vi "Three Chart Temple.vi"(8 "error in (no error)":errorcluster caption="错误输入（无错误）") -> (0 "error out":errorcluster caption="错误输出")   [LabVIEW 2015]
doc: "该连续测量范例项目在队列消息处理器模板的基础上实现。\n\n事件处理循环负责按用户界面操作生成对应的消息。\n\n消息处理循环负责对事件处理循环或其他消息生成的消息进行处理。其中还包括用于采集和记录消息处理循环的子VI，以及用于更新图表的循环。"
uses:
  Settings/Settings.ctl
  Acquisition/Hardware Configuration.ctl
  Logging/Logging Configuration.ctl
  Motor Control/Hardware Configuration.ctl
  controls/UI Data.ctl
  controls/UI State.ctl
  support/Message Queue/Enqueue Message (Single).vi
  <vilib>/Utility/error.llb/Error Cluster From Error Code.vi
  <vilib>/ErrorRing/Error Ring.xnode
  Acquisition/Acquisition.lvlib
  Logging/Logging.lvlib
  Settings/Settings.lvlib
  support/User Event - Stop/User Event - Stop.lvlib
  support/Message Queue/Message Queue.lvlib
  Motor Control/Motor Control.lvlib
panel:
  out "XY Graph":cluster{"Y":dbl[], "Y":dbl[]}[](graph) caption="XY图"
  out "XY Graph 2":cluster{"Y":dbl[], "Y":dbl[]}[](graph) caption="XY图"
  out "XY Graph 3":cluster{"Y":dbl[], "Y":dbl[]}[](graph) caption="XY图"
  in  "清零":bool
  in  "读取":bool
  out "模拟通道5":dbl
  out "模拟通道4":dbl
  out "模拟通道3":dbl
  out "模拟通道2":dbl
  out "模拟通道1":dbl
  out "模拟通道0":dbl
  out "角度":dbl
  in  "计算":bool
  in  "Start":bool caption="开始"
  in  "Stop":bool caption="停止"
  out "Status":string caption="状态"
  in  "Exit":bool caption="退出"
  # "测量项目"
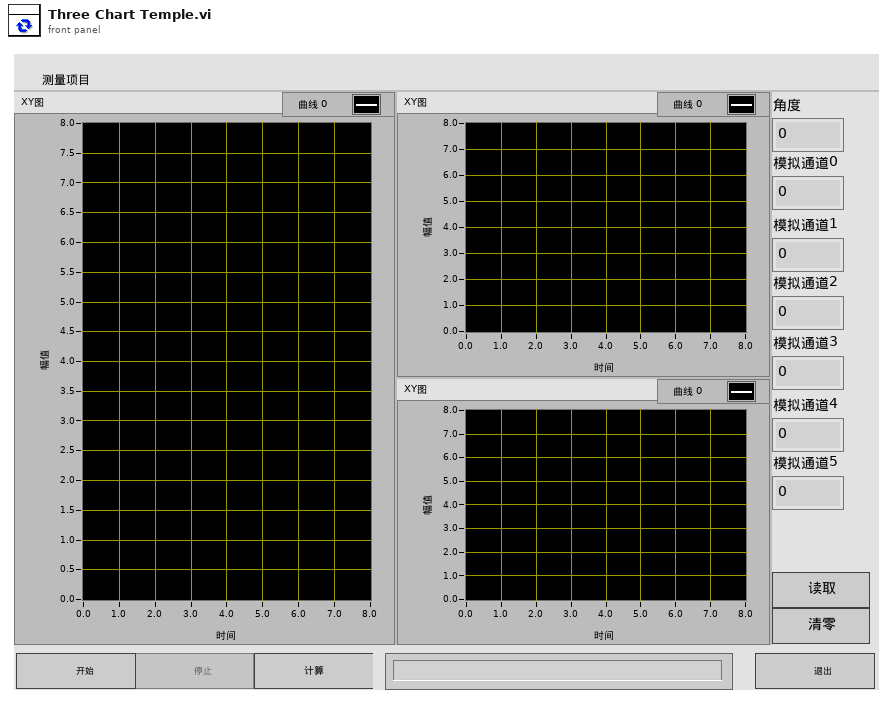
[diagram p1: front panel]
types:
  T1 = typedef "Motor Control.lvlib/电机转动逻辑1.ctl" = cluster{"反转判断条件1":T2, "停止判断条件1":T3}
  T2 = typedef "Motor Control.lvlib/反转判断条件1.ctl" = cluster{"传感器序号":i32, "条件":enum16{"小于", "大于", "等于"}, "值":dbl, "条件判断时间间隔":i32}
  T3 = typedef "Motor Control.lvlib/停止判断条件1.ctl" = cluster{"角度传感器序号":i32, "正转/反转":enum16{"正转", "反转"}, "反转次数":i32, "停止角度":dbl, "停止角度误差范围":dbl}
  T4 = typedef "UI State.ctl" = enum16{"Idle", "Acquiring and Logging", "Waiting for Exit", "Waiting for Exit (Acq Stopped)", "Waiting for Exit (Log Stopped)", "Waiting for Stop", "Waiting for Stop (Acq Stopped)", "Waiting for Stop (Log Stopped)"}
  T5 = typedef "UI Data.ctl" = cluster{"Start Ref":refnum<vi>, "Stop Ref":refnum<vi>, "calculate Ref":refnum<vi>, "Status Ref":refnum<vi>, "Exit Ref":refnum<vi>, "Data Ref":refnum<vi>, "read Ref":refnum<vi>, "clean Ref":refnum<vi>}
  T6 = typedef "Settings.lvlib/Settings.ctl" = cluster{"Hardware Configuration":T7, "Logging Configuration":T8, "电机设置":T9, "啮合测试电机转动逻辑":T1, "功能测试电机转动逻辑":T1, "力提特性电机转动逻辑":T1}
  T7 = typedef "Acquisition.lvlib/Hardware Configuration.ctl" = cluster{"电压读取设置":cluster{"DAQmx Channel":tag, "Max Input":dbl, "Min Input":dbl, "Sample Rate":dbl, "Sample Number":i32, "DAQmx Task":refnum<k21>}, "角度传感器设置":cluster{"counter":tag, "units":i32, "分辨率":i32, "初始角度":dbl, "DecodingType":i32, "A相端口":tag, "B相端口":tag, "task in":refnum<k21>}}
  T8 = typedef "Logging.lvlib/Logging Configuration.ctl" = cluster{"Log File Base Path":path, "电压传感器转换率":dbl[], "电压传感器本底":dbl[]}
  T9 = typedef "Motor Control.lvlib/Hardware Configuration.ctl" = cluster{"counter":tag, "方向端口":tag, "当前方向":bool, "频率":dbl, "DAQmx Task":refnum<k21>}
  T10 = typedef "Message Queue.lvlib/All Message Queues.ctl" = cluster{"UI":refnum<queue>, "Acquisition":refnum<queue>, "Logging":refnum<queue>, "MotorCtrl":refnum<queue>, "plot logic":refnum<queue>}
  T11 = typedef "Logging.lvlib/计算类型.ctl" = enum16{"啮合", "退回", "功能", "力特性"}
  T12 = enum8{"Enabled", "Disabled", "Disabled and Grayed Out"}
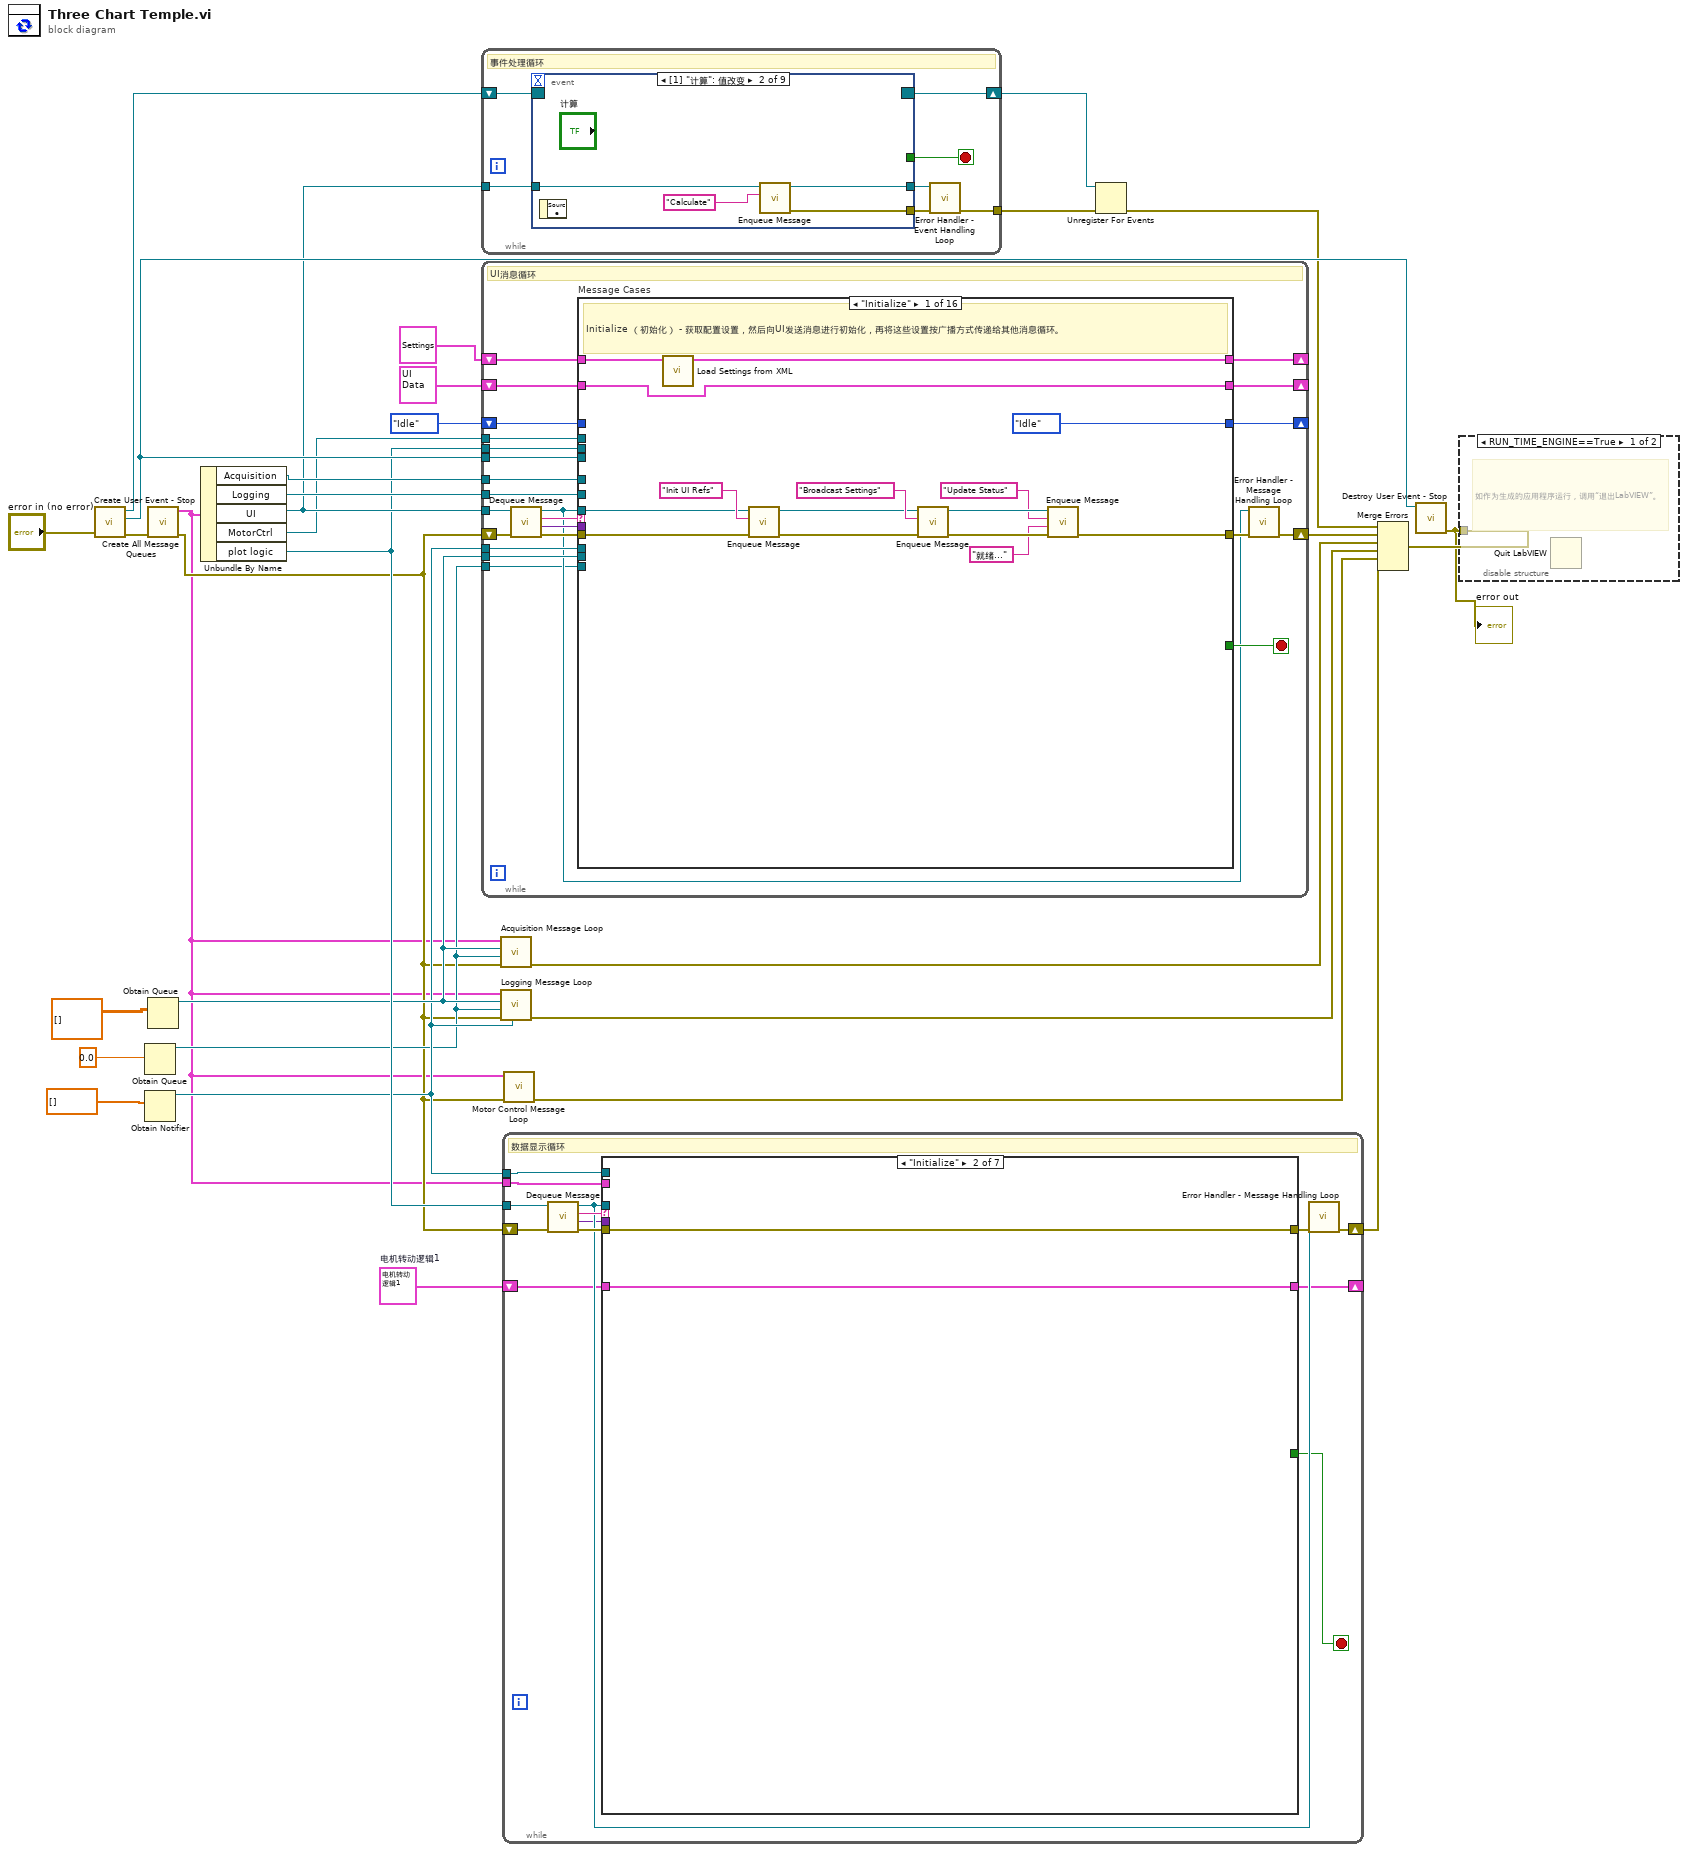
[diagram p0: block diagram]
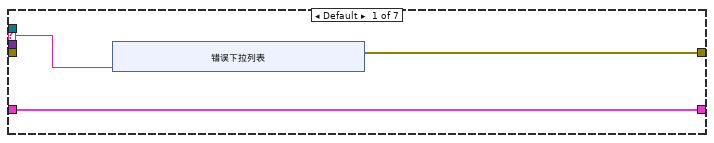
[diagram p3: hidden frame]
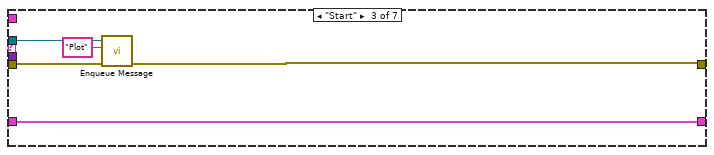
[diagram p4: hidden frame]
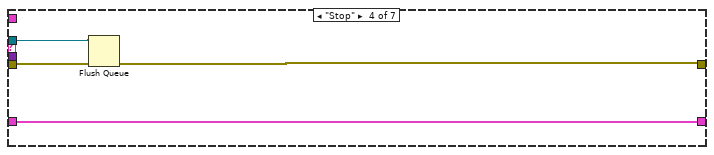
[diagram p5: hidden frame]
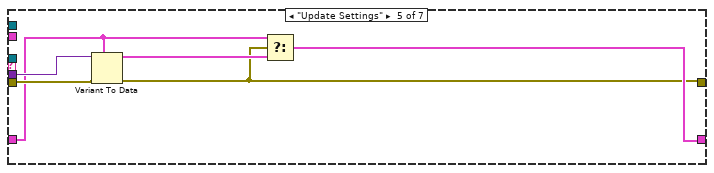
[diagram p6: hidden frame]
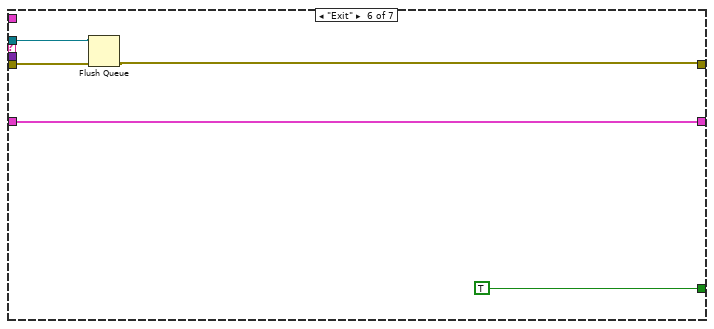
[diagram p7: hidden frame]
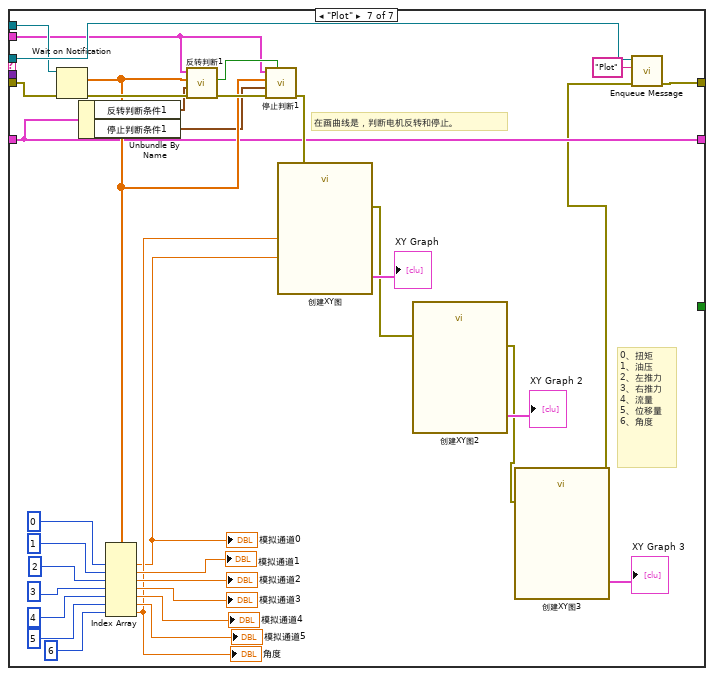
[diagram p8: hidden frame]
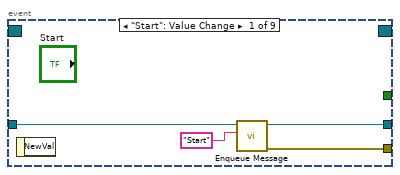
[diagram p9: hidden frame]
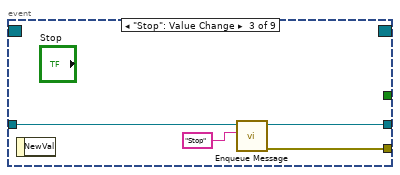
[diagram p10: hidden frame]
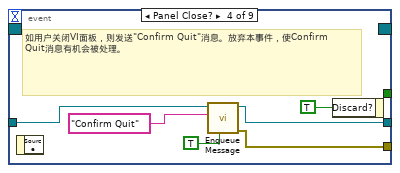
[diagram p11: hidden frame]
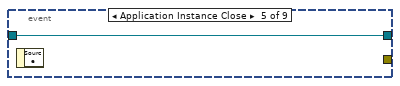
[diagram p12: hidden frame]
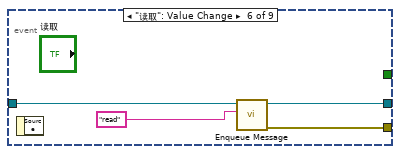
[diagram p13: hidden frame]
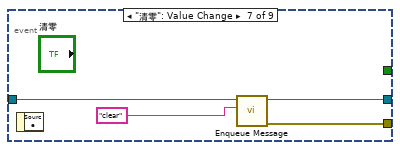
[diagram p14: hidden frame]
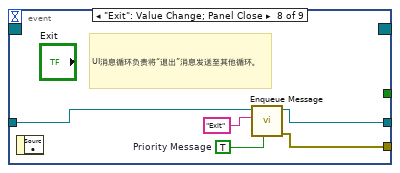
[diagram p15: hidden frame]
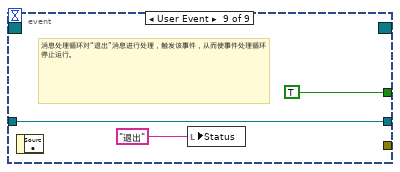
[diagram p16: hidden frame]
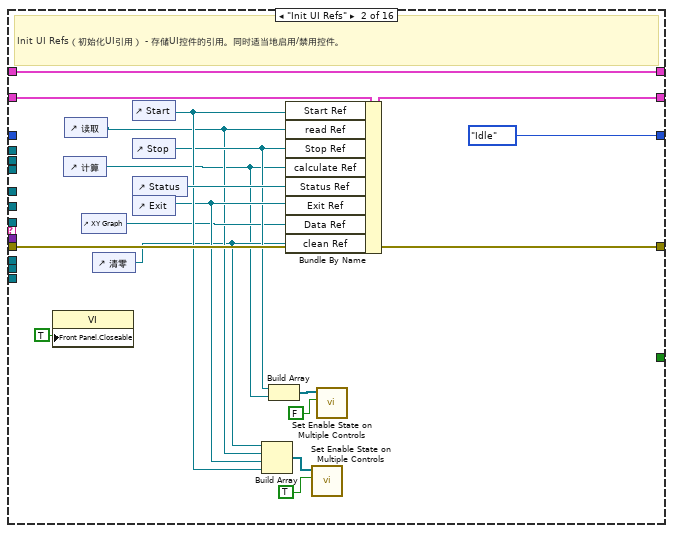
[diagram p17: hidden frame]
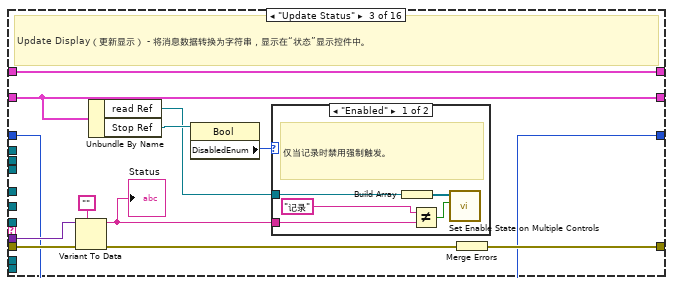
[diagram p18: hidden frame]
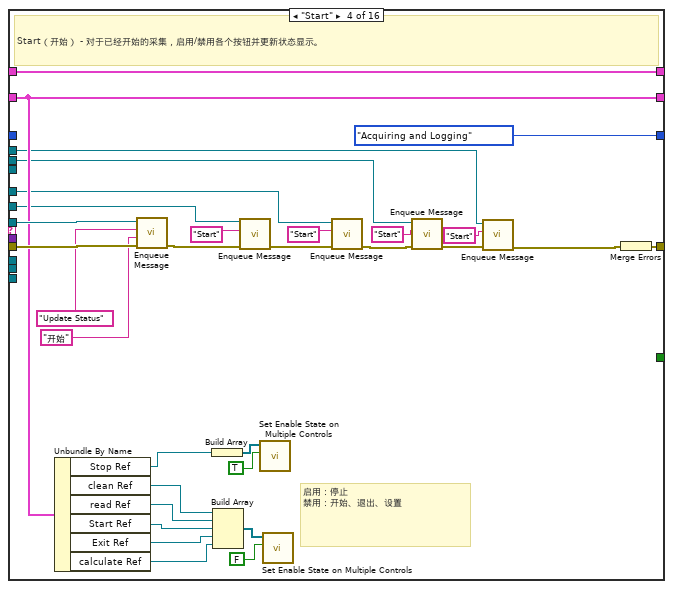
[diagram p20: hidden frame]
diagram:
  w3 = T1 {"反转判断条件1"={"传感器序号"=0, "条件"=enum."小于", "值"=0.0, "条件判断时间间隔"=0}, "停止判断条件1"={"角度传感器序号"=0, "正转/反转"=enum."正转", "反转次数"=0, "停止角度"=0.0, "停止角度误差范围"=0.0}}  # 电机转动逻辑1
  n1 = call "Create User Event - Stop.vi"("error in (no error)"="error in (no error)") -> ("error out"=w25:errorcluster, "User Event - Stop"=w27:refnum<user-event>, "Stop Event Registration Refnum"=w28:refnum<event-registration>)  [unwired: 8 in]
  n2 = Obtain Queue(element data type=0.0) -> (queue out=w8:refnum<queue>)  [unwired: 4 in, 2 out]
  n3 = Obtain Notifier(notification data type=dbl[] []) -> (notifier out=w10:refnum<notifier>)  [unwired: 3 in, 2 out]
  n4 = call "Create All Message Queues.vi"("error in (no error)"=w25) -> ("error out"=w7:errorcluster, "Message Queues out"=w4:T10)  [unwired: 9 in]
  n5 = Obtain Queue(element data type=dbl[][] []) -> (queue out=w11:refnum<queue>)  [unwired: 4 in, 2 out]
  n6 = Unbundle By Name(w4) -> ("Acquisition"=w19:refnum<queue>, "Logging"=w18:refnum<queue>, "UI"=w17:refnum<queue>, "MotorCtrl"=w15:refnum<queue>, "plot logic"=w14:refnum<queue>)
  n7 = while {
    tunnel: w17 -> [w37]
    tunnel: [w32] -> w30
    shift-right: [w36] -> w21
    shift-left: w28 -> [w38]
    stop <- w35 stop-if-true
    # "事件处理循环"
    n8 = event shown="[1] \"计算\": 值改变" {
      selector: w38 -> [_ _ _ _ _ _ _ _ _]
      dyn-events: [_ _ _ _ _ _ _ _ _] -> w36
      timeout: _ -> [_ _ _ _ _ _ _ _ _]
      tunnel: [_ _ _ _ _ _ _ _ TRUE ("Discard?")] -> w35
      tunnel: w37 -> [w40 w45 w49 w56 w57 w59 w63 w67 w71]
      tunnel: [w42 w44 w48 w51 _ w61 w65 w70 _] -> w33
      tunnel: [w39 w43 w47 w52 w57 w58 w62 w66 w71] -> w34
      event "Start": Value Change {
        n9 = event-data() -> ()  [unwired: 1 in, 1 out]
        n10 = call-poly "Enqueue Message.vi"("Message"="Start", "Message Queue"=w40) -> ("error out"=w42:errorcluster, "dup Message Queue"=w39:refnum<queue>)  [unwired: 8 in]
      }
      event "计算": Value Change {
        n11 = event-data() -> ()  [unwired: 1 in, 1 out]
        n12 = call-poly "Enqueue Message.vi"("Message"="Calculate", "Message Queue"=w45) -> ("error out"=w44:errorcluster, "dup Message Queue"=w43:refnum<queue>)  [unwired: 8 in]
      }
      event "Stop": Value Change {
        n13 = event-data() -> ()  [unwired: 1 in, 1 out]
        n14 = call-poly "Enqueue Message.vi"("Message"="Stop", "Message Queue"=w49) -> ("error out"=w48:errorcluster, "dup Message Queue"=w47:refnum<queue>)  [unwired: 8 in]
      }
      event Panel Close? {
        # "如用户关闭VI面板，则发送\"Confirm Quit\"消息。放弃本事件，使Confirm Quit消息有机会被处理。"
        n15 = event-data() -> ()  [unwired: 1 in, 1 out]
        n16 = call-poly "Enqueue Message.vi"("Priority Message? (F)"=TRUE, "Message"="Confirm Quit", "Message Queue"=w56) -> ("error out"=w51:errorcluster, "dup Message Queue"=w52:refnum<queue>)  [unwired: 7 in]
        n17 = event-data("Discard?"=TRUE) -> ()  [unwired: 1 in, 1 out]
      }
      event Application Instance Close {
        n18 = event-data() -> ()  [unwired: 1 in, 1 out]
      }
      event "读取": Value Change {
        n19 = event-data() -> ()  [unwired: 1 in, 1 out]
        n20 = call-poly "Enqueue Message.vi"("Message"="read", "Message Queue"=w59) -> ("error out"=w61:errorcluster, "dup Message Queue"=w58:refnum<queue>)  [unwired: 8 in]
      }
      event "清零": Value Change {
        n21 = event-data() -> ()  [unwired: 1 in, 1 out]
        n22 = call-poly "Enqueue Message.vi"("Message"="clear", "Message Queue"=w63) -> ("error out"=w65:errorcluster, "dup Message Queue"=w62:refnum<queue>)  [unwired: 8 in]
      }
      event "Exit": Value Change; Panel Close {
        w68 = TRUE  # Priority Message
        # "UI消息循环负责将“退出”消息发送至其他循环。"
        n23 = event-data() -> ()  [unwired: 1 in, 1 out]
        n24 = call-poly "Enqueue Message.vi"("Priority Message? (F)"=w68, "Message"="Exit", "Message Queue"=w67) -> ("error out"=w70:errorcluster, "dup Message Queue"=w66:refnum<queue>)  [unwired: 7 in]
      }
      event User Event {
        # "消息处理循环对“退出”消息进行处理，触发该事件，从而使事件处理循环停止运行。"
        n25 = event-data() -> ()  [unwired: 1 in, 1 out]
        n26 = local write "Status"("退出" ("Exit String")) -> ()
      }
    }
    n27 = call "Error Handler - Event Handling Loop.vi"("error in (no error)"=w33, "Message Queue"=w34) -> ("dup error in"=w32:errorcluster)  [unwired: 8 in, 1 out]
  }
  n28 = while {
    tunnel: w17 -> [w90]
    tunnel: w27 -> [w95]
    shift-right: [w80] -> w31
    shift-left: w7 -> [w94]
    shift-right: [w89] -> _
    shift-left: T6 {"Hardware Configuration"={"电压读取设置"={"DAQmx Channel"="", "Max Input"=0.0, "Min Input"=0.0, "Sample Rate"=0.0, "Sample Number"=0, "DAQmx Task"=""}, "角度传感器设置"={"counter"="Dev1/ctr0", "units"=10146, "分辨率"=0, "初始角度"=0.0, "DecodingType"=10092, "A相端口"="/Dev1/PFI8", "B相端口"="/Dev1/PFI8", "task in"=""}}, "Logging Configuration"={"Log File Base Path"=path "", "电压传感器转换率"=[], "电压传感器本底"=[]}, "电机设置"={"counter"="Dev1/ctr0", "方向端口"="", "当前方向"=FALSE, "频率"=0.0, "DAQmx Task"=""}, "啮合测试电机转动逻辑"={"反转判断条件1"={"传感器序号"=0, "条件"=enum."小于", "值"=0.0, "条件判断时间间隔"=0}, "停止判断条件1"={"角度传感器序号"=0, "正转/反转"=enum."正转", "反转次数"=0, "停止角度"=0.0, "停止角度误差范围"=0.0}}, "功能测试电机转动逻辑"={"反转判断条件1"={"传感器序号"=0, "条件"=enum."小于", "值"=0.0, "条件判断时间间隔"=0}, "停止判断条件1"={"角度传感器序号"=0, "正转/反转"=enum."正转", "反转次数"=0, "停止角度"=0.0, "停止角度误差范围"=0.0}}, "力提特性电机转动逻辑"={"反转判断条件1"={"传感器序号"=0, "条件"=enum."小于", "值"=0.0, "条件判断时间间隔"=0}, "停止判断条件1"={"角度传感器序号"=0, "正转/反转"=enum."正转", "反转次数"=0, "停止角度"=0.0, "停止角度误差范围"=0.0}}} ("Settings") -> [w88]
    shift-right: [w86] -> _
    shift-left: T5 {"Start Ref"=refnum, "Stop Ref"=refnum, "calculate Ref"=refnum, "Status Ref"=refnum, "Exit Ref"=refnum, "Data Ref"=refnum, "read Ref"=refnum, "clean Ref"=refnum} ("Measurement UI Controls") -> [w87]
    tunnel: w19 -> [w85]
    tunnel: w18 -> [w84]
    tunnel: w10 -> [w83]
    tunnel: w11 -> [w82]
    shift-right: [w77] -> _
    shift-left: UI_State."Idle" ("UI State") -> [w78]
    tunnel: w15 -> [w74]
    tunnel: w14 -> [w75]
    tunnel: w8 -> [w76]
    stop <- w96 stop-if-true
    # "UI消息循环"
    n29 = call "Dequeue Message.vi"("error in (no error)"=w94, "Message Queue"=w90) -> ("error out"=w93:errorcluster, "Message Data"=w91:variant, "Message"=w92:string, "dup Message Queue"=w79:refnum<queue>)  [unwired: 6 in]
    n30 = case "Message Cases" shown="\"Initialize\"" w92 {
      selector: w92 -> [_ _ _ _ _ _ _ _ _ _ _ _ _ _ _ w381]
      tunnel: w79 -> [w101 _ _ w176 _ w216 w220 w245 _ w293 w308 w318 w356 _ _ _]
      tunnel: w93 -> [w100 w129 w140 w175 w182 w215 w222 w247 w270 w295 w312 w317 w363 w370 w375 _]
      tunnel: [w107 w129 w141 w177 w185 w217 w221 w246 w287 w290 w303 w316 w364 w369 w379 w382] -> w81
      tunnel: [_ _ _ _ _ _ _ _ _ _ _ _ TRUE _ _ _] -> w96
      tunnel: w91 -> [_ _ w139 _ _ _ _ _ _ _ w311 _ _ _ _ _]
      tunnel: w95 -> [_ _ _ _ _ _ _ _ _ _ _ _ w362 _ _ _]
      tunnel: [w110 w128 w136 w174 w184 w214 w226 w251 w285 w292 w314 w321 w360 w368 w378 w384] -> w89
      tunnel: w88 -> [w111 w128 w136 w174 w184 w214 w226 w251 w285 w296 w314 w321 w360 w368 w378 w384]
      tunnel: w87 -> [w103 w127 w135 w171 w183 w211 w225 w250 w282 w289 w313 w320 w359 w367 w377 w383]
      tunnel: [w103 w126 w135 w171 w183 w211 w225 w250 w282 w289 w313 w320 w359 w367 w377 w383] -> w86
      tunnel: w85 -> [_ _ _ w159 _ w199 _ _ w281 _ _ _ w358 _ _ _]
      tunnel: w84 -> [_ _ _ w161 w179 w202 _ _ w280 _ _ _ w357 _ w373 _]
      tunnel: w83 -> [_ _ _ _ _ _ _ _ _ _ _ _ w355 _ _ _]
      tunnel: w82 -> [_ _ _ _ _ _ _ _ _ _ _ _ w352 _ _ _]
      tunnel: w78 -> [_ _ w130 _ w178 w197 w224 w249 w279 w288 w302 w319 _ w366 w376 w380]
      tunnel: [UI_State."Idle" ("UI State") UI_State."Idle" ("UI State") w130 UI_State."Acquiring and Logging" ("UI State") w178 w196 w223 w248 w279 w288 w302 w315 UI_State."Idle" ("UI State") w366 w376 w380] -> w77
      tunnel: w76 -> [_ _ _ _ _ _ _ _ _ _ _ _ w347 _ _ _]
      tunnel: w75 -> [_ _ _ w153 _ w189 _ _ w274 _ _ _ w346 _ _ _]
      tunnel: w74 -> [_ _ _ w149 _ w187 _ _ w277 _ _ _ w345 _ _ _]
      frame "Initialize" {
        # "Initialize （初始化） - 获取配置设置，然后向UI发送消息进行初始化，再将这些设置按广播方式传递给其他消息循环。"
        n31 = call "Load Settings from XML.vi"("Settings in"=w111) -> ("Settings out"=w110:T6)  [unwired: 9 in, 1 out]
        n32 = call-poly "Enqueue Message.vi"("error in (no error)"=w100, "Message"="Init UI Refs", "Message Queue"=w101) -> ("error out"=w98:errorcluster, "dup Message Queue"=w99:refnum<queue>)  [unwired: 7 in]
        n33 = call-poly "Enqueue Message.vi"("error in (no error)"=w98, "Message"="Broadcast Settings", "Message Queue"=w99) -> ("error out"=w109:errorcluster, "dup Message Queue"=w108:refnum<queue>)  [unwired: 7 in]
        n34 = call-poly "Enqueue Message.vi"("error in (no error)"=w109, "Message Data"="就绪..." ("Ready..."), "Message"="Update Status", "Message Queue"=w108) -> ("error out"=w107:errorcluster)  [unwired: 6 in, 1 out]
      }
      frame "Init UI Refs" {
        # "Init UI Refs（初始化UI引用） - 存储UI控件的引用。同时适当地启用/禁用控件。"
        n35 = property class="VI"("Front Panel.Closeable"=TRUE ("Front Panel Window:Closeable")) -> ()  [unwired: 2 in, 2 out]
        n36 = control-ref of="计算"() -> (w112:refnum<vi>)
        n37 = control-ref of="读取"() -> (w114:refnum<vi>)
        n38 = control-ref of="XY Graph"() -> (w115:refnum<vi>)
        n39 = control-ref of="清零"() -> (w113:refnum<vi>)
        n40 = control-ref of="Start"() -> (w122:refnum<vi>)
        n41 = control-ref of="Stop"() -> (w118:refnum<vi>)
        n42 = control-ref of="Status"() -> (w123:refnum<vi>)
        n43 = control-ref of="Exit"() -> (w119:refnum<vi>)
        n44 = Build Array(w113, w114, w119, w122) -> (w121:refnum<vi>[])
        n45 = Build Array(w118, w112) -> (w117:refnum<vi>[])
        n46 = Bundle By Name(cluster=w127, "Start Ref"=w122, "read Ref"=w114, "Stop Ref"=w118, "calculate Ref"=w112, "Status Ref"=w123, "Exit Ref"=w119, "Data Ref"=w115, "clean Ref"=w113) -> (w126:T5)
        n47 = call "Set Enable State on Multiple Controls.vi"("Enable?"=TRUE, "Controls"=w121) -> ()  [unwired: 10 in]
        n48 = call "Set Enable State on Multiple Controls.vi"("Enable?"=FALSE, "Controls"=w117) -> ()  [unwired: 10 in]
      }
      frame "Update Status" {
        # "Update Display（更新显示） - 将消息数据转换为字符串，显示在“状态”显示控件中。"
        n49 = Variant To Data(error in=w140, type="", Variant=w139) -> (data=w132:string, error out=w137:errorcluster)
        "Status" <- w132
        n50 = Unbundle By Name(w135) -> ("read Ref"=w131:refnum<vi>, "Stop Ref"=w134:refnum<vi>)
        n51 = property class="Bool"(reference=w134) -> ("DisabledEnum"=w133:T12)  [unwired: 1 in, 2 out]
        n52 = case shown="\"Enabled\"" w133 {
          tunnel: w132 -> [w144 _]
          tunnel: w131 -> [w145 _]
          frame "Enabled" {
            # "仅当记录时禁用强制触发。"
            n53 = Build Array(w145) -> (w146:refnum<vi>[])
            n54 = Not Equal?(x="记录" ("Logging"), y=w144) -> (x != y?=w142:bool)
            n55 = call "Set Enable State on Multiple Controls.vi"("Enable?"=w142, "Controls"=w146) -> ()  [unwired: 10 in]
          }
          frame "Disabled", Default {
          }
        }
        n56 = Merge Errors(w137) -> (w141:errorcluster)
      }
      frame "Start" {
        # "启用：停止\n禁用：开始、退出、设置"
        # "Start（开始） - 对于已经开始的采集，启用/禁用各个按钮并更新状态显示。"
        n57 = Unbundle By Name(w171) -> ("Stop Ref"=w154:refnum<vi>, "clean Ref"=w155:refnum<vi>, "read Ref"=w156:refnum<vi>, "Start Ref"=w166:refnum<vi>, "Exit Ref"=w165:refnum<vi>, "calculate Ref"=w164:refnum<vi>)
        n58 = call-poly "Enqueue Message.vi"("error in (no error)"=w175, "Message Data"="开始" ("Waiting for trigger"), "Message"="Update Status", "Message Queue"=w176) -> ("error out"=w163:errorcluster)  [unwired: 6 in, 1 out]
        n59 = Build Array(w154) -> (w168:refnum<vi>[])
        n60 = Build Array(w155, w156, w166, w165, w164) -> (w169:refnum<vi>[])
        n61 = call-poly "Enqueue Message.vi"("error in (no error)"=w163, "Message"="Start", "Message Queue"=w161) -> ("error out"=w160:errorcluster)  [unwired: 7 in, 1 out]
        n62 = call "Set Enable State on Multiple Controls.vi"("Enable?"=TRUE, "Controls"=w168) -> ()  [unwired: 10 in]
        n63 = call "Set Enable State on Multiple Controls.vi"("Enable?"=FALSE, "Controls"=w169) -> ()  [unwired: 10 in]
        n64 = call-poly "Enqueue Message.vi"("error in (no error)"=w160, "Message"="Start", "Message Queue"=w159) -> ("error out"=w151:errorcluster)  [unwired: 7 in, 1 out]
        n65 = call-poly "Enqueue Message.vi"("error in (no error)"=w151, "Message"="Start", "Message Queue"=w153) -> ("error out"=w150:errorcluster)  [unwired: 7 in, 1 out]
        n66 = call-poly "Enqueue Message.vi"("error in (no error)"=w150, "Message"="Start", "Message Queue"=w149) -> ("error out"=w147:errorcluster)  [unwired: 7 in, 1 out]
        n67 = Merge Errors(w147) -> (w177:errorcluster)
      }
      frame "Force Trigger" {
        # "Force Trigger（强制触发） - 发送消息至记录消息循环，开始记录。"
        n68 = call-poly "Enqueue Message.vi"("error in (no error)"=w182, "Message"="Force Trigger", "Message Queue"=w179) -> ("error out"=w181:errorcluster)  [unwired: 7 in, 1 out]
        n69 = Merge Errors(w181) -> (w185:errorcluster)
      }
      frame "Stop" {
        # "停止画图、电机、记录，最后停止采集。"
        # "启用：开始、退出、设置\n禁用：停止"
        # "停止－对于已经停止的采集，启用/禁用各个按钮并更新状态显示。"
        n70 = Unbundle By Name(w211) -> ("Stop Ref"=w193:refnum<vi>, "read Ref"=w194:refnum<vi>, "clean Ref"=w195:refnum<vi>, "Start Ref"=w206:refnum<vi>, "Exit Ref"=w205:refnum<vi>, "calculate Ref"=w204:refnum<vi>)
        n71 = call-poly "Enqueue Message.vi"("error in (no error)"=w215, "Message Data"="就绪..." ("Ready..."), "Message"="Update Status", "Message Queue"=w216) -> ("error out"=w192:errorcluster)  [unwired: 6 in, 1 out]
        n72 = Build Array(w194, w195, w206, w205, w204) -> (w209:refnum<vi>[])
        n73 = Build Array(w193) -> (w208:refnum<vi>[])
        n74 = call "Set Enable State on Multiple Controls.vi"("Enable?"=TRUE, "Controls"=w209) -> ()  [unwired: 10 in]
        n75 = call "Set Enable State on Multiple Controls.vi"("Enable?"=FALSE, "Controls"=w208) -> ()  [unwired: 10 in]
        n76 = call-poly "Enqueue Message.vi"("error in (no error)"=w192, "Message"="Stop", "Message Queue"=w189) -> ("error out"=w191:errorcluster)  [unwired: 7 in, 1 out]
        n77 = call-poly "Enqueue Message.vi"("error in (no error)"=w191, "Message"="Stop", "Message Queue"=w187) -> ("error out"=w190:errorcluster)  [unwired: 7 in, 1 out]
        n78 = call-poly "Enqueue Message.vi"("error in (no error)"=w190, "Message"="Stop", "Message Queue"=w202) -> ("error out"=w201:errorcluster)  [unwired: 7 in, 1 out]
        n79 = case shown="默认" w197 {
          selector: w197 -> [_ w219]
          tunnel: [UI_State."Waiting for Stop" ("UI State") w219] -> w196
          frame Default {
          }
          frame "Waiting for Exit" {
          }
        }
        n80 = call-poly "Enqueue Message.vi"("error in (no error)"=w201, "Message"="Stop", "Message Queue"=w199) -> ("error out"=w200:errorcluster)  [unwired: 7 in, 1 out]
        n81 = Merge Errors(w200) -> (w217:errorcluster)
      }
      frame "Acquisition Stopped" {
        # "此处代码用于确定采集停止时采取何种操作。"
        n82 = case shown="\"Waiting for Stop (Log Stopped)\"" w224 {
          selector: w224 -> [w228 _ _ _ _]
          tunnel: [w228 UI_State."Waiting for Exit (Acq Stopped)" ("UI State") UI_State."Waiting for Stop (Acq Stopped)" ("UI State") UI_State."Idle" ("UI State") UI_State."Idle" ("UI State")] -> w223
          tunnel: w222 -> [w227 w229 w231 w237 w243]
          tunnel: [w227 w229 w231 w236 w242] -> w221
          tunnel: w220 -> [_ _ _ w235 w241]
          frame Default {
          }
          frame "Waiting for Exit", "Waiting for Exit (Acq Stopped)" {
          }
          frame "Waiting for Stop", "Waiting for Stop (Acq Stopped)" {
          }
          frame "Waiting for Exit (Log Stopped)" {
            # "如果正在等待退出且记录已结束，“采集停止”消息表示应退出。"
            n83 = call-poly "Enqueue Message.vi"("Priority Message? (F)"=TRUE, "error in (no error)"=w237, "Message"="Exit", "Message Queue"=w235) -> ("error out"=w236:errorcluster)  [unwired: 6 in, 1 out]
          }
          frame "Waiting for Stop (Log Stopped)" {
            # "当前状态为等待停止时，如已停止记录，则收到\"Acquisition Stopped\"消息时即可停止。"
            n84 = call-poly "Enqueue Message.vi"("error in (no error)"=w243, "Message Data"="Ready..." ("Message"), "Message"="Update Status", "Message Queue"=w241) -> ("error out"=w242:errorcluster)  [unwired: 6 in, 1 out]
          }
        }
      }
      frame "Logging Stopped" {
        # "此处代码用于确定记录停止时采取何种操作。"
        n85 = case shown="\"Waiting for Stop (Acq Stopped)\"" w249 {
          selector: w249 -> [w253 _ _ _ _]
          tunnel: [w253 UI_State."Waiting for Exit (Log Stopped)" ("UI State") UI_State."Waiting for Stop (Log Stopped)" ("UI State") UI_State."Idle" ("UI State") UI_State."Idle" ("UI State")] -> w248
          tunnel: w247 -> [w252 w254 w256 w262 w268]
          tunnel: [w252 w254 w256 w261 w267] -> w246
          tunnel: w245 -> [_ _ _ w260 w266]
          frame Default {
          }
          frame "Waiting for Exit", "Waiting for Exit (Log Stopped)" {
          }
          frame "Waiting for Stop", "Waiting for Stop (Log Stopped)" {
          }
          frame "Waiting for Exit (Acq Stopped)" {
            # "如果正在等待退出且采集已结束，“记录停止”消息表示应退出。"
            n86 = call-poly "Enqueue Message.vi"("Priority Message? (F)"=TRUE, "error in (no error)"=w262, "Message"="Exit", "Message Queue"=w260) -> ("error out"=w261:errorcluster)  [unwired: 6 in, 1 out]
          }
          frame "Waiting for Stop (Acq Stopped)" {
            # "如果正在等待停止且采集已结束，“记录停止”消息表示应停止。"
            n87 = call-poly "Enqueue Message.vi"("error in (no error)"=w268, "Message Data"="Ready..." ("Message"), "Message"="Update Status", "Message Queue"=w266) -> ("error out"=w267:errorcluster)  [unwired: 6 in, 1 out]
          }
        }
      }
      frame "Broadcast settings" {
        w273 = "Update Settings" ("Message")
        # "向“记录和采集”消息队列发送“更新设置”消息。"
        n88 = Unbundle By Name(w285) -> ("Hardware Configuration"=w284:T7, "Logging Configuration"=w283:T8, "电机设置"=w276:T9, "啮合测试电机转动逻辑"=w272:T1)
        n89 = call-poly "Enqueue Message.vi"("error in (no error)"=w270, "Message Data"=w284, "Message"=w273, "Message Queue"=w281) -> ("error out"=w286:errorcluster)  [unwired: 6 in, 1 out]
        n90 = call-poly "Enqueue Message.vi"("error in (no error)"=w286, "Message Data"=w283, "Message"=w273, "Message Queue"=w280) -> ("error out"=w278:errorcluster)  [unwired: 6 in, 1 out]
        n91 = call-poly "Enqueue Message.vi"("error in (no error)"=w278, "Message Data"=w276, "Message"=w273, "Message Queue"=w277) -> ("error out"=w275:errorcluster)  [unwired: 6 in, 1 out]
        n92 = call-poly "Enqueue Message.vi"("error in (no error)"=w275, "Message Data"=w272, "Message"=w273, "Message Queue"=w274) -> ("error out"=w271:errorcluster)  [unwired: 6 in, 1 out]
        n93 = Merge Errors(w271, w270) -> (w287:errorcluster)
      }
      frame "Launch Settings Dialog" {
        # "用户单击“设置”按钮时，启动设置对话框。"
        n94 = call "Settings Dialog.vi"("error in (no error)"=w295, "Settings in"=w296) -> ("error out"=w291:errorcluster, "Cancelled?"=w294:bool, "Settings out"=w292:T6)  [unwired: 6 in, 1 out]
        n95 = case shown="假" w294 {
          tunnel: w293 -> [w300 _]
          tunnel: w291 -> [w299 w301]
          tunnel: [w298 w301] -> w290
          frame False {
            n96 = call-poly "Enqueue Message.vi"("error in (no error)"=w299, "Message"="Broadcast Settings", "Message Queue"=w300) -> ("error out"=w298:errorcluster)  [unwired: 7 in, 1 out]
          }
          frame True {
          }
        }
      }
      frame "Error" {
        # "Error - 检查错误消息数据及其响应。该消息由应用程序各循环结束处的“错误处理”VI发送。"
        n97 = Variant To Data(error in=w312, type=errorcluster {"status"=FALSE, "code"=0, "source"=""} ("error out"), Variant=w311) -> (data=w309:errorcluster, error out=w305:errorcluster)
        n98 = call <vilib>:"Simple Error Handler.vi"("error in (no error)"=w309) -> ()  [unwired: 4 in, 5 out]
        n99 = call-poly "Enqueue Message.vi"("Priority Message? (F)"=TRUE, "Message"="Exit", "Message Queue"=w308) -> ("error out"=w304:errorcluster)  [unwired: 7 in, 1 out]
        n100 = Merge Errors(w304, w305) -> (w303:errorcluster)
      }
      frame "Confirm Quit" {
        # "Confirm Quit - 该消息用于确认用户是否需要退出应用程序。"
        n101 = case shown="\"Acquiring and Logging\"" w319 {
          tunnel: w318 -> [w326 w332]
          tunnel: w317 -> [w325 w330]
          tunnel: [w322 w329] -> w316
          tunnel: [UI_State."Idle" ("UI State") w328] -> w315
          frame Default {
            # "如收到'Confirm Quit'消息时系统处于空闲状态，则不需要弹出确认提示。"
            n102 = call-poly "Enqueue Message.vi"("Priority Message? (F)"=TRUE, "error in (no error)"=w325, "Message"="Exit", "Message Queue"=w326) -> ("error out"=w322:errorcluster)  [unwired: 6 in, 1 out]
          }
          frame "Acquiring and Logging" {
            n103 = Two Button Dialog(message="采集仍在执行中，是否确定退出？" ("Confirm Quit Message"), 1:"否" ("No"), 2:"是" ("Yes")) -> (T button?=w331:bool)
            n104 = case shown="真" w331 {
              tunnel: w332 -> [_ w342]
              tunnel: w330 -> [w336 w341]
              tunnel: [w336 w340] -> w329
              tunnel: [UI_State."Acquiring and Logging" ("UI State") UI_State."Waiting for Exit" ("UI State")] -> w328
              frame False {
                # "用户不希望退出。"
              }
              frame True {
                n105 = call-poly "Enqueue Message.vi"("error in (no error)"=w341, "Message"="Stop", "Message Queue"=w342) -> ("error out"=w340:errorcluster)  [unwired: 7 in, 1 out]
              }
            }
          }
        }
      }
      frame "Exit" {
        w343 = TRUE ("Priority Message? (F)")
        w344 = "Exit" ("Message")
        # "不必检查错误输出。采集和记录队列可能已被释放。"
        # "停止VI。"
        # "Exit（退出）－触发用户事件，使“事件处理”循环停止运行。同时向“采集和记录”循环发送“退出”消息。"
        n106 = Release Queue(queue=w356, error in (no error)=w363) -> (error out=w354:errorcluster)  [unwired: 1 in, 2 out]
        n107 = call "Fire User Event - Stop.vi"("User Event - Stop"=w362) -> ("error out"=w361:errorcluster)  [unwired: 10 in]
        n108 = Release Notifier(notifier=w355, error in (no error)=w354) -> (error out=w353:errorcluster)  [unwired: 1 in, 2 out]
        n109 = Release Queue(queue=w352, error in (no error)=w353) -> (error out=w349:errorcluster)  [unwired: 1 in, 2 out]
        n110 = call-poly "Enqueue Message.vi"("Priority Message? (F)"=TRUE, "Message"=w344, "Message Queue"=w358) -> ()  [unwired: 7 in, 2 out]
        n111 = Release Queue(queue=w347, error in (no error)=w349) -> (error out=w348:errorcluster)  [unwired: 1 in, 2 out]
        n112 = call-poly "Enqueue Message.vi"("Priority Message? (F)"=w343, "Message"=w344, "Message Queue"=w357) -> ()  [unwired: 7 in, 2 out]
        n113 = call-poly "Enqueue Message.vi"("Priority Message? (F)"=w343, "Message"=w344, "Message Queue"=w346) -> ()  [unwired: 7 in, 2 out]
        n114 = call-poly "Enqueue Message.vi"("Priority Message? (F)"=w343, "Message"=w344, "Message Queue"=w345) -> ()  [unwired: 7 in, 2 out]
        n115 = Merge Errors(w361, w348) -> (w364:errorcluster)
      }
      frame "---Copy This Frame---" {
        # "如需创建新消息，可创建该帧的副本。在副本中，将本注释更改为对应消息的注释。"
        n116 = Merge Errors(w370) -> (w369:errorcluster)
      }
      frame "Calculate" {
        # "发指令让记录线程执行计算，传入相应的计算类型。"
        # "如需创建新消息，可创建该帧的副本。在副本中，将本注释更改为对应消息的注释。"
        n117 = call-poly "Enqueue Message.vi"("error in (no error)"=w375, "Message Data"=计算类型."啮合" ("计算类型"), "Message"="Calculate", "Message Queue"=w373) -> ("error out"=w374:errorcluster)  [unwired: 6 in, 1 out]
        n118 = Merge Errors(w374) -> (w379:errorcluster)
      }
      frame Default {
        # "如得到的消息未经任何分支定义，则运行“默认”分支。输出程序错误。"
        n119 = xnode "错误下拉列表"("参数 0"=w381) -> ("错误输出"=w382:errorcluster)
      }
    }
    n120 = call "Error Handler - Message Handling Loop.vi"("error in (no error)"=w81, "Message Queue"=w79) -> ("dup error in"=w80:errorcluster)  [unwired: 8 in, 1 out]
  }
  n121 = call "Acquisition Message Loop.vi"("error in (no error)"=w7, "Angle Data Queue"=w8, "Analog Data Queue"=w11, "Message Queues"=w4) -> ("error out"=w26:errorcluster)  [unwired: 7 in]
  n122 = call "Logging Message Loop.vi"("数据通知器"=w10, "error in (no error)"=w7, "Angle Data Queue"=w8, "Analog Data Queue"=w11, "Message Queues"=w4) -> ("error out"=w24:errorcluster)  [unwired: 6 in]
  n123 = while "Data Display Loop" {
    tunnel: w10 -> [w397]
    tunnel: w14 -> [w404]
    shift-right: [w399] -> w5
    shift-left: w7 -> [w403]
    tunnel: w4 -> [w395]
    shift-right: [w392] -> _
    shift-left: w3 -> [w393]
    stop <- w396 stop-if-true
    # "数据显示循环"
    n124 = call "Dequeue Message.vi"("error in (no error)"=w403, "Message Queue"=w404) -> ("error out"=w401:errorcluster, "Message Data"=w394:variant, "Message"=w400:string, "dup Message Queue"=w398:refnum<queue>)  [unwired: 6 in]
    n125 = case shown="\"Initialize\"" w400 {
      selector: w400 -> [w406 _ _ _ _ _ _]
      tunnel: [w407 w415 w418 w424 w426 w434 w453] -> w402
      tunnel: w401 -> [_ w415 w421 w425 w430 w436 w467]
      tunnel: w398 -> [_ _ w420 w423 _ w435 w470]
      tunnel: w397 -> [_ _ _ _ _ _ w468]
      tunnel: [_ _ _ _ _ TRUE _] -> w396
      tunnel: w395 -> [_ _ _ _ _ _ w447]
      tunnel: w394 -> [_ _ _ _ w429 _ _]
      tunnel: [w405 w416 w417 w422 w427 w432 w444] -> w392
      tunnel: w393 -> [w405 w416 w417 w422 w428 w432 w444]
      frame Default {
        n126 = xnode "错误下拉列表"("参数 0"=w406) -> ("错误输出"=w407:errorcluster)
      }
      frame "Initialize" {
      }
      frame "Start" {
        n127 = call-poly "Enqueue Message.vi"("error in (no error)"=w421, "Message"="Plot", "Message Queue"=w420) -> ("error out"=w418:errorcluster)  [unwired: 7 in, 1 out]
      }
      frame "Stop" {
        n128 = Flush Queue(queue=w423, error in (no error)=w425) -> (error out=w424:errorcluster)  [unwired: 2 out]
      }
      frame "Update Settings" {
        n129 = Variant To Data(error in=w430, type=w428, Variant=w429) -> (data=w431:T1, error out=w426:errorcluster)
        n130 = Select(t=w428, s=w426, f=w431) -> (s? t:f=w427:T1)
      }
      frame "Exit" {
        n131 = Flush Queue(queue=w435, error in (no error)=w436) -> (error out=w434:errorcluster)  [unwired: 2 out]
      }
      frame "Plot" {
        # "在画曲线是，判断电机反转和停止。"
        # "0、扭矩\n1、油压\n2、左推力\n3、右推力\n4、流量\n5、位移量\n6、角度"
        n132 = Wait on Notification(notifier=w468, error in (no error)=w467) -> (notification=w446:dbl[], error out=w450:errorcluster)  [unwired: 2 in, 2 out]
        n133 = Unbundle By Name(w444) -> ("反转判断条件1"=w443:T2, "停止判断条件1"=w442:T3)
        n134 = Index Array(array=w446, index #1=0 ("索引"), index #2=1 ("索引"), index #3=2 ("索引"), index #4=3 ("索引"), index #5=4 ("索引"), index #6=5 ("索引"), index #7=6 ("索引")) -> (element #1=w451:dbl, element #2=→"模拟通道1":dbl, element #3=→"模拟通道2":dbl, element #4=→"模拟通道3":dbl, element #5=→"模拟通道4":dbl, element #6=→"模拟通道5":dbl, element #7=w452:dbl)
        "角度" <- w452
        "模拟通道0" <- w451
        n135 = call "反转判断1.vi"("error in (no error)"=w450, "反转判断条件1"=w443, "传感器数据"=w446, "Message Queues"=w447) -> ("error out"=w449:errorcluster, "反转"=w448:bool)  [unwired: 6 in]
        n136 = call "停止判断1.vi"("反转？"=w448, "error in (no error)"=w449, "反转判断条件1"=w442, "传感器数据"=w446, "Message Queues"=w447) -> ("error out"=w445:errorcluster)  [unwired: 6 in]
        n137 = call "创建XY图"("error in (no error)"=w445, "Y Input"=w451, "X Input"=w452) -> ("error out"=w439:errorcluster, "XY Graph"=→"XY Graph":cluster{"X":dbl[], "Y":dbl[]}[])  [unwired: 7 in]
        n138 = call "创建XY图2"("error in (no error)"=w439) -> ("error out"=w438:errorcluster, "XY Graph"=→"XY Graph 2":cluster{"X":dbl[], "Y":dbl[]}[])  [unwired: 9 in]
        n139 = call "创建XY图3"("error in (no error)"=w438) -> ("error out"=w437:errorcluster, "XY Graph"=→"XY Graph 3":cluster{"X":dbl[], "Y":dbl[]}[])  [unwired: 9 in]
        n140 = call-poly "Enqueue Message.vi"("error in (no error)"=w437, "Message"="Plot", "Message Queue"=w470) -> ("error out"=w453:errorcluster)  [unwired: 7 in, 1 out]
      }
    }
    n141 = call "Error Handler - Message Handling Loop.vi"("error in (no error)"=w402, "Message Queue"=w398) -> ("dup error in"=w399:errorcluster)  [unwired: 8 in, 1 out]
  }
  n142 = call "Motor Control Message Loop.vi"("error in (no error)"=w7, "Message Queues"=w4) -> ("error out"=w6:errorcluster)  [unwired: 9 in]
  n143 = Unregister For Events(event registration refnum=w21, error in=w30) -> (error out=w22:errorcluster)
  n144 = Merge Errors(w22, w31, w26, w24, w6, w5) -> (w29:errorcluster)
  n145 = call "Destroy User Event - Stop.vi"("error in (no error)"=w29, "User Event - Stop"=w27) -> ("error out"=w2:errorcluster)  [unwired: 9 in]
  "error out" <- w2
  n146 = disable-structure shown="RUN_TIME_ENGINE==True" {
    disable-tunnel: w2 -> [_ _]
    frame condition #0 {
      # "如作为生成的应用程序运行，调用“退出LabVIEW”。"
      n147 = Quit LabVIEW() -> ()  [unwired: 1 in]
    }
    frame condition #1 (active) {
    }
  }
